vi "EnQ Sample.vi"(8 "error in (no error)":errorcluster, 10 "Sample.lvclass":refnum<class "Sample.lvclass">, 11 "Preparation Line in":refnum<class "Preparation Line.lvclass">) -> (0 "error out":errorcluster, 3 "Preparation Line out":refnum<class "Preparation Line.lvclass">)   [LabVIEW 2015, in "cRIO-Carbondioxide.lvlib" / "CO2-Actor.lvlib" / "Preparation Line.lvclass"]
uses:
  Preparation Line.lvclass
  subs/Sample/Sample.lvclass
  Preparation Line.lvclass/Preparation Line.ctl
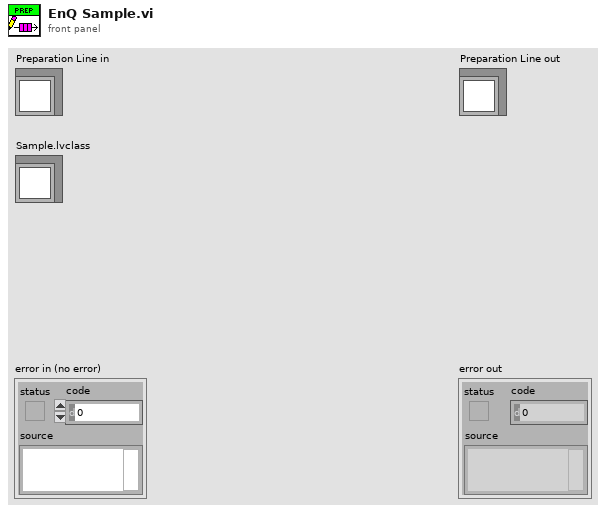
[diagram p1: front panel]
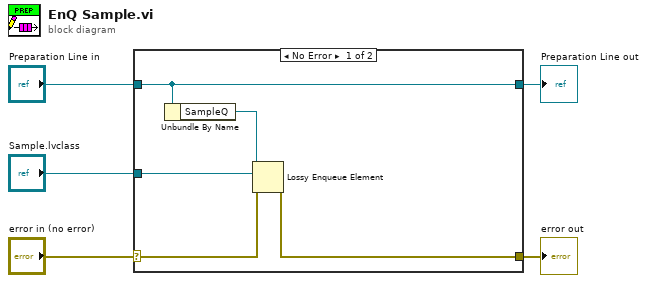
[diagram p0: block diagram]
diagram:
  n1 = case shown="No Error" "error in (no error)" {
    selector: "error in (no error)" -> [w7 w11]
    tunnel: [w6 w11] -> w4
    tunnel: [w10 w12] -> w2
    tunnel: "Preparation Line in" -> [w10 w12]
    tunnel: "Sample.lvclass" -> [w9 _]
    frame No Error {
      n2 = Unbundle By Name(w10) -> ("SampleQ"=w8:refnum<queue>)
      n3 = Lossy Enqueue Element(queue=w8, element=w9, error in (no error)=w7) -> (error out=w6:errorcluster)  [unwired: 3 out]
    }
    frame Error {
    }
  }
  "error out" <- w4
  "Preparation Line out" <- w2
